vi "WorkAsCan.vi"() -> (0 "VCI_CAN_OBJ 2":T1={"ID"=0, "TimeStamp"=0, "TimeFlag"=0, "SendType"=2, "RemoteFlag"=0, "ExternFlag"=0, "DataLen"=0, "Data 0"=0, "Data 1"=1, "Data 2"=0, "Data 3"=0, "Data 4"=0, "Data 5"=0, "Data 6"=0, "Data 7"=0, "Reserved 0"=0, "Reserved 1"=0, "Reserved 2"=0})   [LabVIEW 2014]
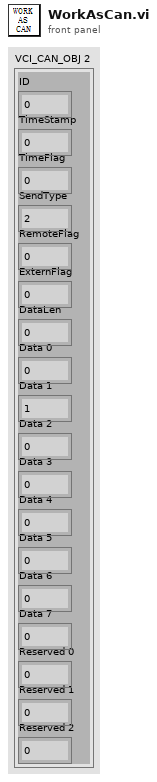
[diagram p1: front panel]
types:
  T1 = cluster{"ID":u32, "TimeStamp":u32, "TimeFlag":u8, "SendType":u8, "RemoteFlag":u8, "ExternFlag":u8, "DataLen":u8, "Data 0":u8, "Data 1":u8, "Data 2":u8, "Data 3":u8, "Data 4":u8, "Data 5":u8, "Data 6":u8, "Data 7":u8, "Reserved 0":u8, "Reserved 1":u8, "Reserved 2":u8}
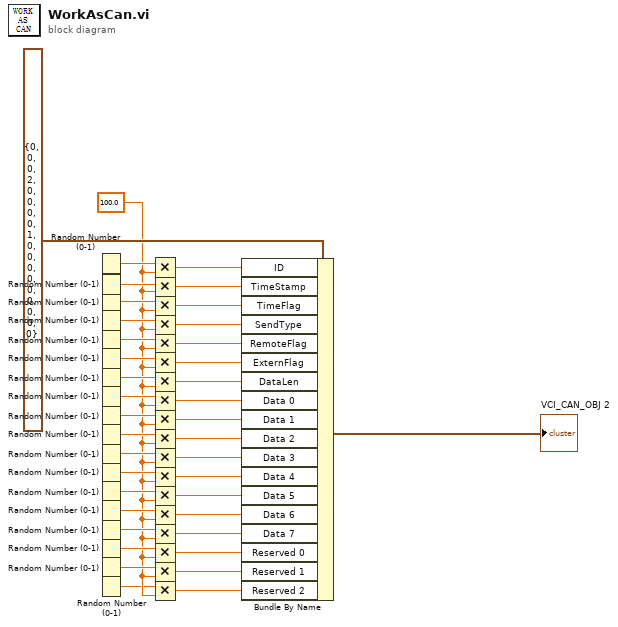
[diagram p0: block diagram]
diagram:
  w2 = 100.0
  n1 = Random Number (0-1)() -> (number: 0 to 1=w37:dbl)
  n2 = Random Number (0-1)() -> (number: 0 to 1=w18:dbl)
  n3 = Random Number (0-1)() -> (number: 0 to 1=w17:dbl)
  n4 = Random Number (0-1)() -> (number: 0 to 1=w16:dbl)
  n5 = Random Number (0-1)() -> (number: 0 to 1=w15:dbl)
  n6 = Random Number (0-1)() -> (number: 0 to 1=w14:dbl)
  n7 = Random Number (0-1)() -> (number: 0 to 1=w13:dbl)
  n8 = Random Number (0-1)() -> (number: 0 to 1=w12:dbl)
  n9 = Random Number (0-1)() -> (number: 0 to 1=w11:dbl)
  n10 = Random Number (0-1)() -> (number: 0 to 1=w10:dbl)
  n11 = Random Number (0-1)() -> (number: 0 to 1=w9:dbl)
  n12 = Random Number (0-1)() -> (number: 0 to 1=w8:dbl)
  n13 = Random Number (0-1)() -> (number: 0 to 1=w7:dbl)
  n14 = Random Number (0-1)() -> (number: 0 to 1=w6:dbl)
  n15 = Random Number (0-1)() -> (number: 0 to 1=w5:dbl)
  n16 = Random Number (0-1)() -> (number: 0 to 1=w4:dbl)
  n17 = Random Number (0-1)() -> (number: 0 to 1=w3:dbl)
  n18 = Random Number (0-1)() -> (number: 0 to 1=w1:dbl)
  n19 = Multiply(x=w37, y=w2) -> (x*y=w36:dbl)
  n20 = Multiply(x=w18, y=w2) -> (x*y=w35:dbl)
  n21 = Multiply(x=w17, y=w2) -> (x*y=w34:dbl)
  n22 = Multiply(x=w16, y=w2) -> (x*y=w33:dbl)
  n23 = Multiply(x=w15, y=w2) -> (x*y=w32:dbl)
  n24 = Multiply(x=w14, y=w2) -> (x*y=w31:dbl)
  n25 = Multiply(x=w13, y=w2) -> (x*y=w30:dbl)
  n26 = Multiply(x=w12, y=w2) -> (x*y=w29:dbl)
  n27 = Multiply(x=w11, y=w2) -> (x*y=w28:dbl)
  n28 = Multiply(x=w10, y=w2) -> (x*y=w27:dbl)
  n29 = Multiply(x=w9, y=w2) -> (x*y=w26:dbl)
  n30 = Multiply(x=w8, y=w2) -> (x*y=w25:dbl)
  n31 = Multiply(x=w7, y=w2) -> (x*y=w24:dbl)
  n32 = Multiply(x=w6, y=w2) -> (x*y=w23:dbl)
  n33 = Multiply(x=w5, y=w2) -> (x*y=w22:dbl)
  n34 = Multiply(x=w4, y=w2) -> (x*y=w21:dbl)
  n35 = Multiply(x=w3, y=w2) -> (x*y=w20:dbl)
  n36 = Multiply(x=w1, y=w2) -> (x*y=w19:dbl)
  n37 = Bundle By Name(cluster=T1 {"ID"=0, "TimeStamp"=0, "TimeFlag"=0, "SendType"=2, "RemoteFlag"=0, "ExternFlag"=0, "DataLen"=0, "Data 0"=0, "Data 1"=1, "Data 2"=0, "Data 3"=0, "Data 4"=0, "Data 5"=0, "Data 6"=0, "Data 7"=0, "Reserved 0"=0, "Reserved 1"=0, "Reserved 2"=0} ("VCI_CAN_OBJ 2"), "ID"=w36, "TimeStamp"=w35, "TimeFlag"=w34, "SendType"=w33, "RemoteFlag"=w32, "ExternFlag"=w31, "DataLen"=w30, "Data 0"=w29, "Data 1"=w28, "Data 2"=w27, "Data 3"=w26, "Data 4"=w25, "Data 5"=w24, "Data 6"=w23, "Data 7"=w22, "Reserved 0"=w21, "Reserved 1"=w20, "Reserved 2"=w19) -> (→"VCI_CAN_OBJ 2":T1)
